vi "Compass_5843_Reading.vi"(2 "SRV In":string) -> (1 "Heading":cluster{"X":dbl, "Y":dbl, "Z":dbl}, 4 "SRV Out":string="169.254.0.10")   [LabVIEW 2009]
panel:
  out "Reply":string
  # "This LabVIEW item is deprecated.\n\nIt is believed to be unused and will be removed in a future version of SRV."
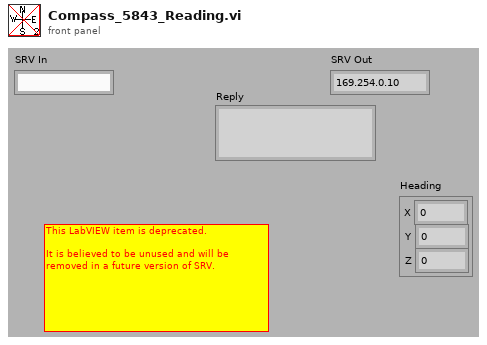
[diagram p1: front panel]
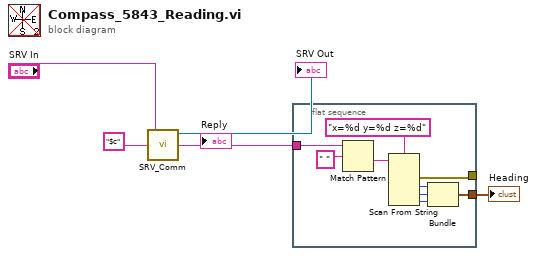
[diagram p0: block diagram]
diagram:
  n1 = call "SRV_Comm.vi"("Command Sent"="$c", "SRV In"="SRV In") -> ("Reply"=w5:string, "SRV Out"=→"SRV Out":refnum<k5>)  [unwired: 1 in, 1 out]
  "Reply" <- w5
  n2 = flat-sequence {
    tunnel: w5 -> [w14]
    tunnel: [w11] -> _
    tunnel: [w6] -> w1
    frame #0 {
      n3 = Match Pattern(string=w14, regular expression=" " ("Command Sent")) -> (after substring=w13:string)  [unwired: 1 in, 3 out]
      n4 = Scan From String(format string="x=%d y=%d z=%d", input string=w13) -> (error out=w11:errorcluster, output 1=w7:i32, output 2=w8:i32, output 3=w9:i32)  [unwired: 5 in, 2 out]
      n5 = Bundle(w7, w8, w9) -> (w6:cluster{i32, i32, i32})  [unwired: 1 in]
    }
  }
  "Heading" <- w1
